vi "DecayTestVerification.vi"(8 "error in":errorcluster, 11 "S1 in":refnum<class "S5.lvclass">) -> (0 "error out":errorcluster, 3 "S1 out":refnum<class "S5.lvclass">)   [LabVIEW 2018, in "S5.lvclass"]
uses:
  S5.lvclass
  S5.lvclass/S5.ctl
  Public Controls/ReportHeader.ctl
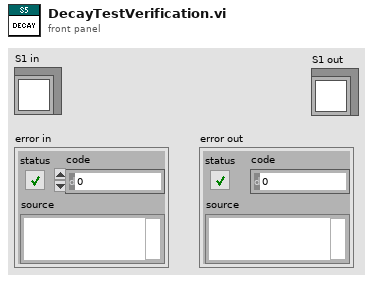
[diagram p1: front panel]
types:
  T1 = typedef "S5.lvclass/ReportHeader.ctl" = string
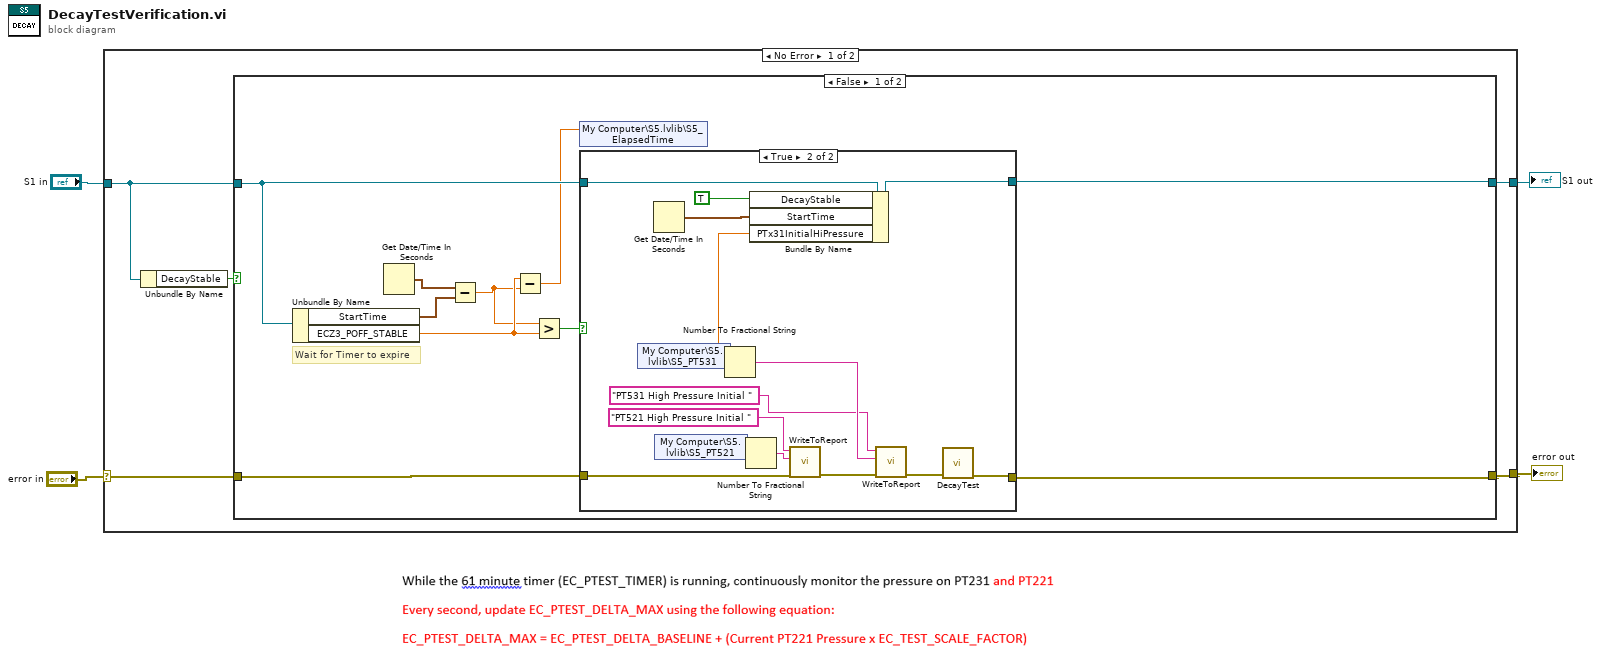
[diagram p0: block diagram]
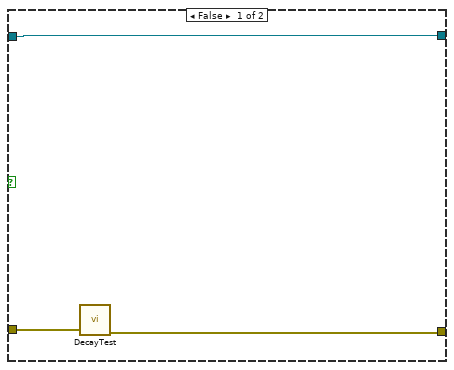
[diagram p2: hidden frame]
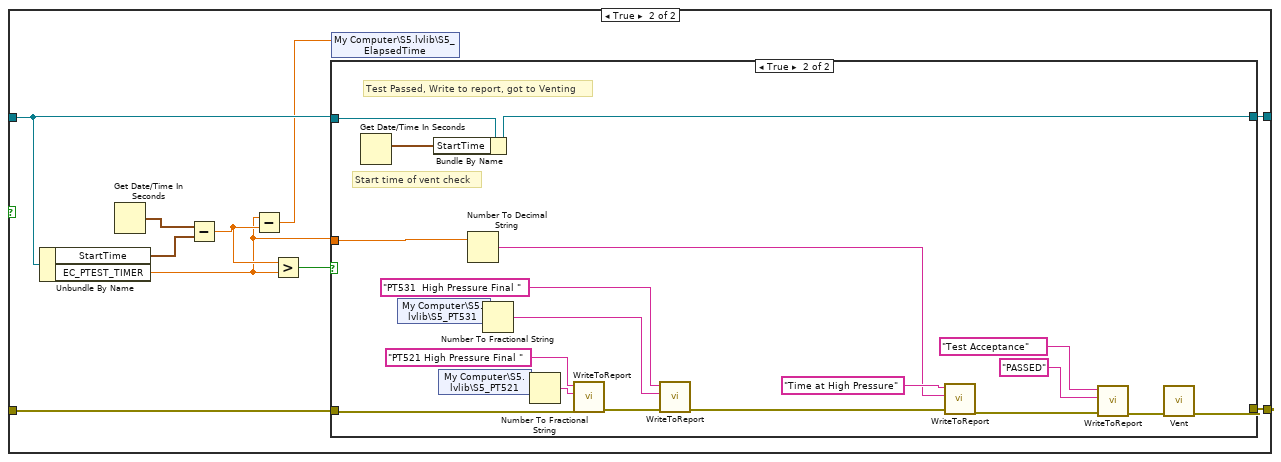
[diagram p3: hidden frame]
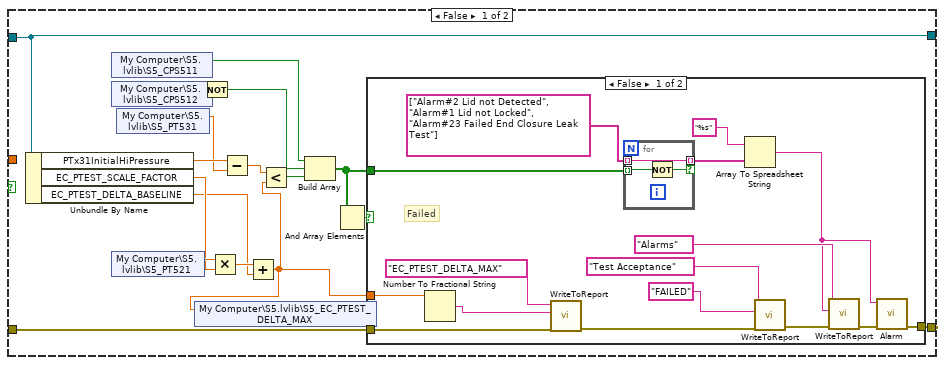
[diagram p4: hidden frame]
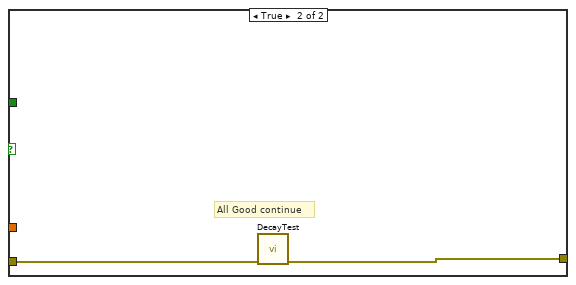
[diagram p5: hidden frame]
diagram:
  n1 = case shown="No Error" "error in" {
    selector: "error in" -> [w9 w106]
    tunnel: [w7 w106] -> w4
    tunnel: "S1 in" -> [w5 w105]
    tunnel: [w8 w105] -> w1
    frame No Error {
      n2 = Unbundle By Name(w5) -> ("DecayStable"=w6:bool)
      n3 = case shown="False" w6 {
        tunnel: w9 -> [w19 w46]
        tunnel: [w18 w45] -> w8
        tunnel: [w17 w44] -> w7
        tunnel: w5 -> [w12 w43]
        frame False {
          # "Wait for Timer to expire"
          n4 = Unbundle By Name(w12) -> ("StartTime"=w14:timestamp, "ECZ3_POFF_STABLE"=w16:dbl)
          n5 = Get Date/Time In Seconds() -> (seconds since 1Jan1904=w13:timestamp)
          n6 = Subtract(x=w13, y=w14) -> (x-y=w15:dbl)
          n7 = Subtract(x=w16, y=w15) -> (x-y=w10:dbl)
          n8 = Greater?(x=w15, y=w16) -> (0:w11:bool)
          n9 = shared-variable "My Computer\\S5.lvlib\\S5_ElapsedTime"(w10) -> ()  [unwired: 1 in, 1 out]
          n10 = case shown="True" w11 {
            tunnel: w19 -> [w22 w26]
            tunnel: [w20 w35] -> w18
            tunnel: [w21 w24] -> w17
            tunnel: w12 -> [w20 w36]
            frame False {
              n11 = call "DecayTest.vi"("error in"=w22) -> ("error out"=w21:errorcluster)  [unwired: 10 in]
            }
            frame True {
              n12 = shared-variable "My Computer\\S5.lvlib\\S5_PT531"() -> (w23:dbl)  [unwired: 1 in, 1 out]
              n13 = Get Date/Time In Seconds() -> (seconds since 1Jan1904=w33:timestamp)
              n14 = shared-variable "My Computer\\S5.lvlib\\S5_PT521"() -> (w31:dbl)  [unwired: 1 in, 1 out]
              n15 = Number To Fractional String(number=w23) -> (F-format string=w29:string)  [unwired: 3 in]
              n16 = Number To Fractional String(number=w31) -> (F-format string=w30:string)  [unwired: 3 in]
              n17 = Bundle By Name(cluster=w36, "DecayStable"=TRUE, "StartTime"=w33, "PTx31InitialHiPressure"=w23) -> (w35:refnum<class "S5.lvclass">)
              n18 = call "WriteToReport.vi"("error in"=w26, "Value"=w30, "Header"="PT521 High Pressure Initial " ("F-format string")) -> ("error out"=w32:errorcluster)  [unwired: 8 in]
              n19 = call "WriteToReport.vi"("error in"=w32, "Value"=w29, "Header"="PT531 High Pressure Initial " ("F-format string")) -> ("error out"=w25:errorcluster)  [unwired: 8 in]
              n20 = call "DecayTest.vi"("error in"=w25) -> ("error out"=w24:errorcluster)  [unwired: 10 in]
            }
          }
        }
        frame True {
          n21 = Unbundle By Name(w43) -> ("StartTime"=w41:timestamp, "EC_PTEST_TIMER"=w37:dbl)
          n22 = Get Date/Time In Seconds() -> (seconds since 1Jan1904=w42:timestamp)
          n23 = Subtract(x=w42, y=w41) -> (x-y=w39:dbl)
          n24 = Subtract(x=w37, y=w39) -> (x-y=w38:dbl)
          n25 = Greater?(x=w39, y=w37) -> (0:w40:bool)
          n26 = case shown="True" w40 {
            tunnel: [w63 w89] -> w44
            tunnel: w46 -> [w62 w97]
            tunnel: w43 -> [w61 w96]
            tunnel: [w61 w91] -> w45
            tunnel: w37 -> [_ w86]
            frame False {
              n27 = Unbundle By Name(w61) -> ("PTx31InitialHiPressure"=w60:dbl, "EC_PTEST_SCALE_FACTOR"=w50:dbl, "EC_PTEST_DELTA_BASELINE"=w48:dbl)
              n28 = shared-variable "My Computer\\S5.lvlib\\S5_CPS511"() -> (w54:bool)  [unwired: 1 in, 1 out]
              n29 = shared-variable "My Computer\\S5.lvlib\\S5_CPS512"() -> (w57:bool)  [unwired: 1 in, 1 out]
              n30 = shared-variable "My Computer\\S5.lvlib\\S5_PT521"() -> (w51:dbl)  [unwired: 1 in, 1 out]
              n31 = shared-variable "My Computer\\S5.lvlib\\S5_PT531"() -> (w59:dbl)  [unwired: 1 in, 1 out]
              n32 = Not(x=w57) -> (.not. x?=w55:bool)
              n33 = Multiply(x=w51, y=w50) -> (x*y=w49:dbl)
              n34 = Subtract(x=w60, y=w59) -> (x-y=w58:dbl)
              n35 = Add(x=w49, y=w48) -> (x+y=w47:dbl)
              n36 = shared-variable "My Computer\\S5.lvlib\\S5_EC_PTEST_DELTA_MAX"(w47) -> ()  [unwired: 1 in, 1 out]
              n37 = Less?(x=w58, y=w47) -> (x < y?=w56:bool)
              n38 = Build Array(w54, w55, w56) -> (w52:bool[])
              n39 = And Array Elements(Boolean array=w52) -> (logical AND=w53:bool)
              n40 = case shown="False" w53 {
                tunnel: [w77 w83] -> w63
                tunnel: w62 -> [w67 w84]
                tunnel: w52 -> [w73 _]
                tunnel: w47 -> [w65 _]
                frame False {
                  # "Failed"
                  n41 = Number To Fractional String(number=w65) -> (F-format string=w64:string)  [unwired: 3 in]
                  n42 = call "WriteToReport.vi"("error in"=w67, "Value"=w64, "Header"=T1 "EC_PTEST_DELTA_MAX") -> ("error out"=w66:errorcluster)  [unwired: 8 in]
                  n43 = for {
                    tunnel: w73 -> [w81] mode=indexing
                    tunnel: string[] ["Alarm#2 Lid not Detected", "Alarm#1 Lid not Locked", "Alarm#23 Failed End Closure Leak Test"] -> [w82] mode=indexing
                    tunnel: [w82] -> w70 mode=indexing if=w80
                    n44 = Not(x=w81) -> (.not. x?=w80:bool)
                  }
                  n45 = Array To Spreadsheet String(array=w70, 3:"%s" ("format string")) -> (spreadsheet string=w69:string)  [unwired: 1 in]
                  n46 = call "WriteToReport.vi"("error in"=w66, "Value"="FAILED", "Header"=T1 "Test Acceptance") -> ("error out"=w75:errorcluster)  [unwired: 8 in]
                  n47 = call "WriteToReport.vi"("error in"=w75, "Value"=w69, "Header"="Alarms") -> ("error out"=w76:errorcluster)  [unwired: 8 in]
                  n48 = call "Alarm.vi"("error in"=w76, "Alarm"=w69) -> ("error out"=w77:errorcluster)  [unwired: 9 in]
                }
                frame True {
                  # "All Good continue"
                  n49 = call "DecayTest.vi"("error in"=w84) -> ("error out"=w83:errorcluster)  [unwired: 10 in]
                }
              }
            }
            frame True {
              # "Test Passed, Write to report, got to Venting"
              # "Start time of vent check"
              n50 = Get Date/Time In Seconds() -> (seconds since 1Jan1904=w90:timestamp)
              n51 = shared-variable "My Computer\\S5.lvlib\\S5_PT531"() -> (w85:dbl)  [unwired: 1 in, 1 out]
              n52 = Bundle By Name(cluster=w96, "StartTime"=w90) -> (w91:refnum<class "S5.lvclass">)
              n53 = shared-variable "My Computer\\S5.lvlib\\S5_PT521"() -> (w102:dbl)  [unwired: 1 in, 1 out]
              n54 = Number To Decimal String(number=w86) -> (decimal integer string=w92:string)  [unwired: 1 in]
              n55 = Number To Fractional String(number=w85) -> (F-format string=w100:string)  [unwired: 3 in]
              n56 = Number To Fractional String(number=w102) -> (F-format string=w101:string)  [unwired: 3 in]
              n57 = call "WriteToReport.vi"("error in"=w97, "Value"=w101, "Header"="PT521 High Pressure Final " ("F-format string")) -> ("error out"=w103:errorcluster)  [unwired: 8 in]
              n58 = call "WriteToReport.vi"("error in"=w103, "Value"=w100, "Header"="PT531  High Pressure Final " ("F-format string")) -> ("error out"=w95:errorcluster)  [unwired: 8 in]
              n59 = call "WriteToReport.vi"("error in"=w95, "Value"=w92, "Header"="Time at High Pressure" ("F-format string")) -> ("error out"=w94:errorcluster)  [unwired: 8 in]
              n60 = call "WriteToReport.vi"("error in"=w94, "Value"="PASSED", "Header"=T1 "Test Acceptance") -> ("error out"=w104:errorcluster)  [unwired: 8 in]
              n61 = call "Vent.vi"("error in"=w104) -> ("error out"=w89:errorcluster)  [unwired: 10 in]
            }
          }
          n62 = shared-variable "My Computer\\S5.lvlib\\S5_ElapsedTime"(w38) -> ()  [unwired: 1 in, 1 out]
        }
      }
    }
    frame Error {
    }
  }
  "error out" <- w4
  "S1 out" <- w1
